vi "Write Cell and Format.vi"(7 "output cluster":cluster{"row":i32, "column":i32}, 8 "error in (no error)":errorcluster, 9 "Data In":dbl format="%#_6f", 10 "format string":string="%0.6f", 11 "NI_report in":refnum<class "NI_report.lvclass">) -> (0 "error out":errorcluster, 3 "NI_report out":refnum<class "NI_report.lvclass">)   [LabVIEW 2016]
uses:
  <vilib>/Utility/NIReport.llb/NI_report.lvclass
  <vilib>/addons/_office/NI_ReportGenerationToolkit.lvlib
  <vilib>/Utility/NIReport.llb/Excel/NI_Excel.lvclass
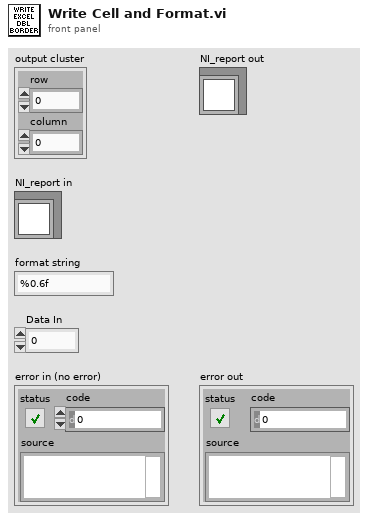
[diagram p1: front panel]
types:
  T1 = cluster{"on/off":bool, "weight":i32, "color":u32}
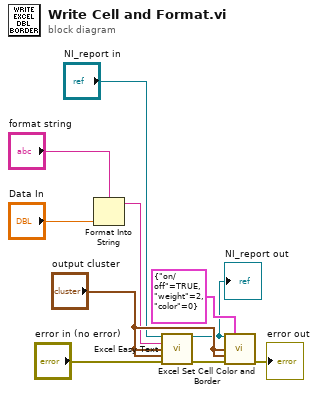
[diagram p0: block diagram]
diagram:
  n1 = Format Into String(format string="format string", "Data In") -> (resulting string=w4:string)  [unwired: 2 in, 1 out]
  n2 = call <vilib>:"Excel Easy Text.vi"("report in"="NI_report in", "text"=w4, "start (-1, -1)"="output cluster", "end (-1, -1)"="output cluster", "error in (no error)"="error in (no error)") -> ("report out"=w8:refnum<class "NI_report.lvclass">, "error out"=w6:errorcluster)  [unwired: 6 in, 3 out]
  "NI_report out" <- w8
  n3 = call <vilib>:"Excel Set Cell Color and Border.vi"("report in"=w8, "inside border"=T1 {"on/off"=TRUE, "weight"=2, "color"=0}, "start (-1, -1)"="output cluster", "end (-1, -1)"="output cluster", "error in (no error)"=w6) -> ("error out"=→"error out":errorcluster)  [unwired: 9 in, 1 out]
